vi "RT_skewMatrix (SubVI).vi"(11 "vector":dbl[](array[numeric])) -> (3 "skew matrix":dbl[][](array[numeric]))   [LabVIEW 2017]
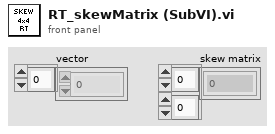
[diagram p1: front panel]
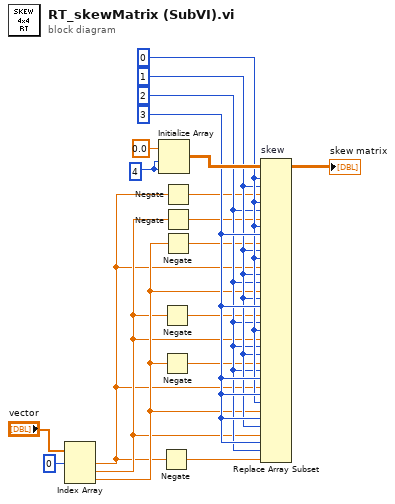
[diagram p0: block diagram]
diagram:
  w14 = 3 ("index (col)")
  w11 = 2 ("index (row)")
  w12 = 1 ("index (col)")
  w13 = 0 ("index (row)")
  w17 = 4 ("dimension size")
  n1 = Index Array(array="vector", index #1=0 ("index")) -> (element #1=w1:dbl, element #2=w2:dbl, element #3=w3:dbl)  [unwired: 2 in]
  n2 = Initialize Array(0.0 ("element"), w17, w17) -> (w15:dbl[][])
  n3 = Negate(x=w1) -> (-x=w4:dbl)
  n4 = Negate(x=w2) -> (-x=w6:dbl)
  n5 = Negate(x=w3) -> (-x=w5:dbl)
  n6 = Negate(x=w1) -> (-x=w9:dbl)
  n7 = Negate(x=w2) -> (-x=w8:dbl)
  n8 = Negate(x=w3) -> (-x=w7:dbl)
  n9 = Replace Array Subset "skew"(array=w15, new element #1=w9, index (row) #1=w13, index (col) #1=w12, new element #2=w8, index (row) #2=w13, index (col) #2=w11, new element #3=w7, index (row) #3=w13, index (col) #3=w14, new element #4=w1, index (row) #4=w12, index (col) #4=w13, new element #5=w3, index (row) #5=w12, index (col) #5=w11, new element #6=w6, index (row) #6=w12, index (col) #6=w14, new element #7=w2, index (row) #7=w11, index (col) #7=w13, new element #8=w5, index (row) #8=w11, index (col) #8=w12, new element #9=w1, index (row) #9=w11, index (col) #9=w14, new element #10=w3, index (row) #10=w14, index (col) #10=w13, new element #11=w2, index (row) #11=w14, index (col) #11=w12, new element #12=w4, index (row) #12=w14, index (col) #12=w11) -> (→"skew matrix":dbl[][])
